vi "PNS zeitlicher Wechsel Filter-Leitung spuelen.vi"(6 "reset":bool, 8 "Takt Leitung":dbl, 9 "Takt Filter":dbl, 11 "Zustand PNS":T1) -> (3 "Zustand PNS":T1)   [LabVIEW 2020, in "PNS.lvlib"]
doc: "von cRIO kopiert und um reset erweitert - sonst beginnt er mit unvollständigen Zeitintervallen !\n#PNStakten\nriw - 30.08.2018"
uses:
  PNS.lvlib
  Funktionstasten/Zustaende.ctl
  Funktionstasten/Funktionstasten.lvlib
  Aktion PNS zeitlicher Wechsel.ctl
  Aktion PNS FGV variabler Taktmerker.ctl
  Seiten/Erweiterte Konfig/Erweiterte Konfig.lvlib
  Seiten/Erweiterte Konfig/FGV PID Aktionen.ctl
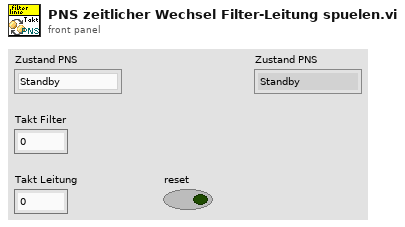
[diagram p1: front panel]
types:
  T1 = typedef "Funktionstasten.lvlib/Zustaende.ctl" = enum16{"Standby", "Pause", "Eco", "Messen", "Kalibrieren", "Spülen Filter", "Spülen Leitung", "Umgebungsluft", "0-Gas", "Cal-Gas", "CG zu PNS", "-------------", "Init 1", "Init 2", "Init 3", "Init 4", "Messen vorbereiten", "Messen durchführen", "Exit"}
  T2 = typedef "PNS.lvlib/Aktion PNS zeitlicher Wechsel.ctl" = enum16{"Zustand vergleichen", "Filterspülen", "Leitung spülen", "Werte einlesen"}
  T3 = typedef "Erweiterte Konfig.lvlib/FGV PID Aktionen.ctl" = enum16{"Lesen", "Schreiben PID", "Schreiben Sonstige", "Dichtheitstest", "Aktionen Dicht.", "Parameter Sensor"}
  T4 = typedef "PNS.lvlib/Aktion PNS FGV variabler Taktmerker.ctl" = enum16{"Lesen", "aktiv", "inaktiv", "Werte schreiben"}
  T5 = typedef "Erweiterte Konfig.lvlib/Sonstige Parameter.ctl" = cluster{"Lüfter langsam":sgl, "Lüfter schnell":sgl, "FT-IR Kühlung Soll":sgl, "FT-IR Kühlung Max":sgl, "Überwachung":T6, "Befüllung aktiv":T7, "Stickstoff Befüllzeit":sgl, "Befüllintervall":sgl, "Kalibrierwert FT-IR":sgl, "Offset Ausgang":sgl, "Offset FT-IR":sgl, "Offset Druck FT-IR":sgl, "Dichtheitstest Zeit":sgl, "Dichtheitstest Abfall":sgl, "Dichtheitstest Umfang":T8, "Offset Umgebung":sgl, "Max Taupunkt":sgl, "Pumpendrehzahl":sgl}
  T6 = typedef "Auswahlfeld.ctl" = u16
  T7 = typedef "LogKonfig.lvlib/Auswahlfeld aktiviert-deaktiviert.ctl" = u16
  T8 = typedef "Erweiterte Konfig.lvlib/Dichtheitstest Umfang.ctl" = u16
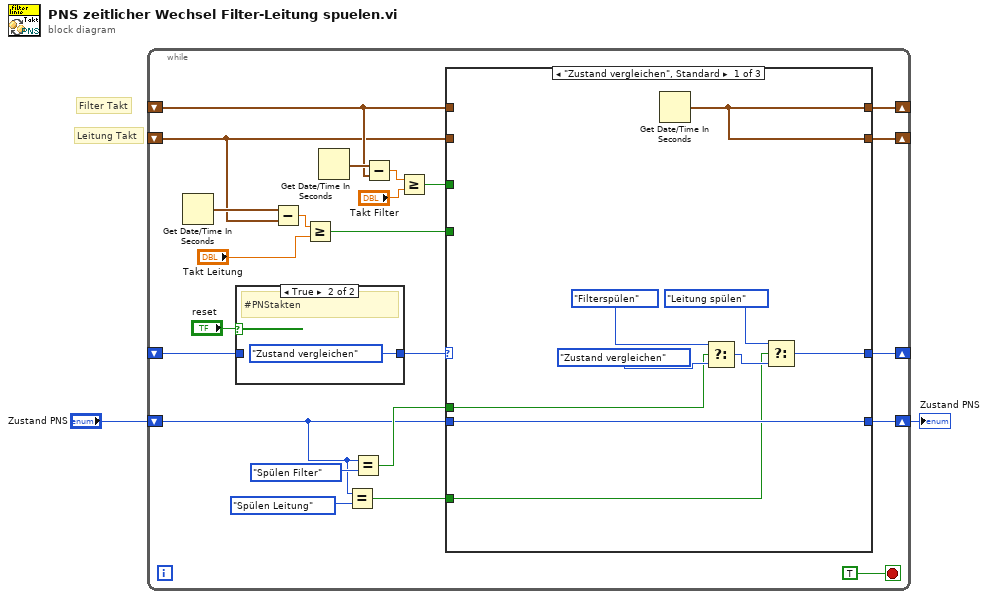
[diagram p0: block diagram]
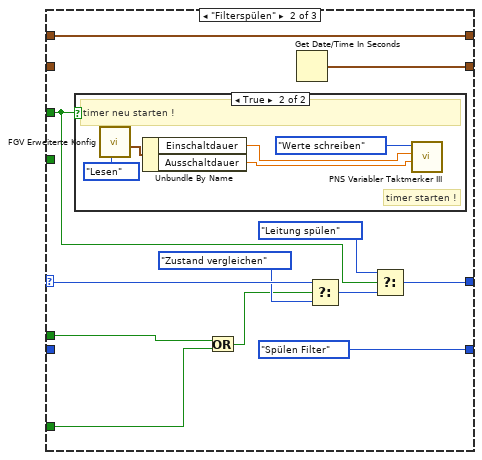
[diagram p3: hidden frame]
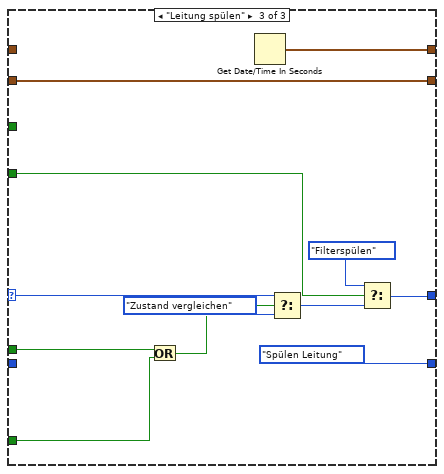
[diagram p5: hidden frame]
diagram:
  # "Leitung Takt"
  # "Filter Takt"
  n1 = while {
    shift-right: [w24] -> w1
    shift-left: "Zustand PNS" -> [w17]
    shift-right: [w21] -> _
    shift-left: _ -> [w4]
    shift-right: [w20] -> _
    shift-left: _ -> [w15]
    shift-right: [w19] -> _
    shift-left: _ -> [w13]
    stop <- TRUE stop-if-true
    n2 = Get Date/Time In Seconds() -> (seconds since 1Jan1904=w14:timestamp)
    n3 = case shown="True" "reset" {
      tunnel: w4 -> [w26 _]
      tunnel: [w26 Aktion_PNS_zeitlicher_Wechsel."Zustand vergleichen" ("Aktion")] -> w3
      frame False {
      }
      frame True {
        # "#PNStakten"
      }
    }
    n4 = Subtract(x=w14, y=w13) -> (x-y=w10:dbl)
    n5 = Greater Or Equal?(x=w10, y="Takt Leitung") -> (x >= y?=w6:bool)
    n6 = Get Date/Time In Seconds() -> (seconds since 1Jan1904=w16:timestamp)
    n7 = Equal?(x=w17, y=Zustaende."Spülen Leitung") -> (x = y?=w8:bool)
    n8 = Equal?(x=w17, y=Zustaende."Spülen Filter") -> (x = y?=w22:bool)
    n9 = Subtract(x=w16, y=w15) -> (x-y=w12:dbl)
    n10 = Greater Or Equal?(x=w12, y="Takt Filter") -> (x >= y?=w7:bool)
    n11 = case shown="\"Zustand vergleichen\", Standard" w3 {
      selector: w3 -> [_ w48 w65]
      tunnel: w17 -> [w36 _ _]
      tunnel: [w36 Zustaende."Spülen Filter" ("Zustand PC") Zustaende."Spülen Leitung" ("Zustand PC")] -> w24
      tunnel: w22 -> [w33 w43 w64]
      tunnel: [w30 w39 w58] -> w21
      tunnel: w15 -> [_ w45 _]
      tunnel: [w32 w45 w61] -> w20
      tunnel: [w32 w44 w60] -> w19
      tunnel: w13 -> [_ _ w60]
      tunnel: w8 -> [w29 w42 w54]
      tunnel: w7 -> [_ w37 _]
      tunnel: w6 -> [_ _ w56]
      frame "Zustand vergleichen", Default {
        n12 = Get Date/Time In Seconds() -> (seconds since 1Jan1904=w32:timestamp)
        n13 = Select(t=Aktion_PNS_zeitlicher_Wechsel."Filterspülen" ("Aktion"), s=w33, f=Aktion_PNS_zeitlicher_Wechsel."Zustand vergleichen" ("Aktion")) -> (s? t:f=w31:T2)
        n14 = Select(t=Aktion_PNS_zeitlicher_Wechsel."Leitung spülen", s=w29, f=w31) -> (s? t:f=w30:T2)
      }
      frame "Filterspülen" {
        n15 = case shown="True" w37 {
          frame False {
          }
          frame True {
            # "timer starten !"
            # "timer neu starten !"
            n16 = call "FGV Erweiterte Konfig.vi"("Aktion"=FGV_PID_Aktionen."Lesen") -> ("Sonstige"=w51:T5)  [unwired: 6 in, 4 out]
            n17 = Unbundle By Name(w51) -> ("Einschaltdauer"=w50:sgl, "Ausschaltdauer"=w49:sgl)
            n18 = call "PNS Variabler Taktmerker III.vi"("Aus in sec."=w49, "Ein in sec."=w50, "Aktion"=Aktion_PNS_FGV_variabler_Taktmerker."Werte schreiben") -> ()  [unwired: 6 in, 3 out]
          }
        }
        n19 = Or(x=w43, y=w42) -> (x .or. y?=w41:bool)
        n20 = Get Date/Time In Seconds() -> (seconds since 1Jan1904=w44:timestamp)
        n21 = Select(t=w48, s=w41, f=Aktion_PNS_zeitlicher_Wechsel."Zustand vergleichen") -> (s? t:f=w40:T2)
        n22 = Select(t=Aktion_PNS_zeitlicher_Wechsel."Leitung spülen", s=w37, f=w40) -> (s? t:f=w39:T2)
      }
      frame "Leitung spülen" {
        n23 = Or(x=w64, y=w54) -> (x .or. y?=w55:bool)
        n24 = Get Date/Time In Seconds() -> (seconds since 1Jan1904=w61:timestamp)
        n25 = Select(t=w65, s=w55, f=Aktion_PNS_zeitlicher_Wechsel."Zustand vergleichen") -> (s? t:f=w59:T2)
        n26 = Select(t=Aktion_PNS_zeitlicher_Wechsel."Filterspülen", s=w56, f=w59) -> (s? t:f=w58:T2)
      }
    }
  }
  "Zustand PNS" <- w1
